vi "Get PC Task List.vi"(8 "error in (no error)":errorcluster) -> (0 "error out":errorcluster, 2 "Tasklist":string)   [LabVIEW 2018, in "BFECC.lvlib" / "BFECC.lvclass"]
uses:
  BFECC.lvclass
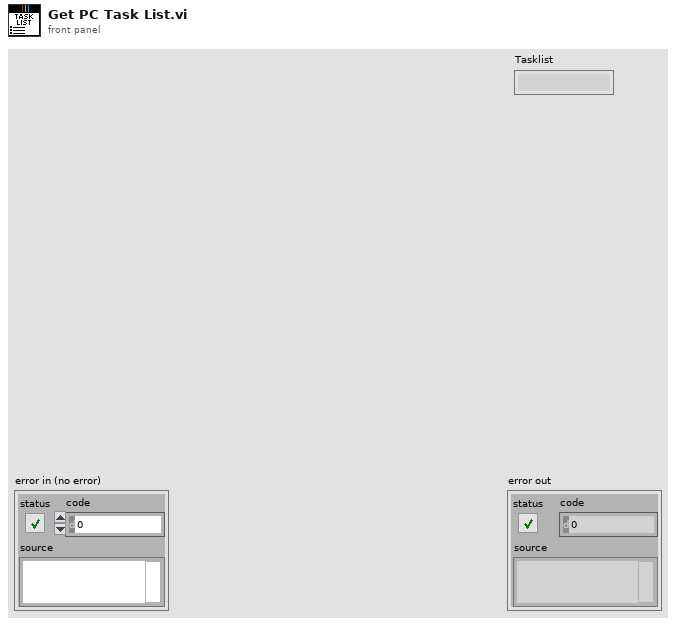
[diagram p1: front panel]
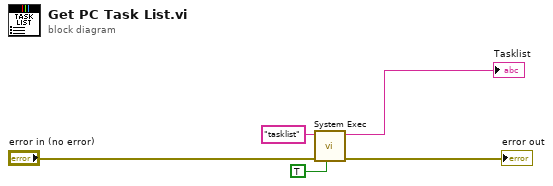
[diagram p0: block diagram]
diagram:
  n1 = call <vilib>:"System Exec.vi"("run minimized? (F)"=TRUE, "error in (no error)"="error in (no error)", "command line"="tasklist") -> ("error out"=→"error out":errorcluster, "standard output"=→"Tasklist":string)  [unwired: 5 in, 2 out]
